vi "Parse Constructor String.vi"(11 "Input":string) -> (0 "error out":errorcluster, 3 "Result":T1)   [LabVIEW 2020, in "Stream.lvlib" / "URLPattern.lvclass"]
uses:
  URLPattern.lvclass
  URL Pattern Init.ctl
  Tokenize Policy.ctl
  Token Type.ctl
  Parser State.ctl
  Is Non-Special Pattern Char.vi
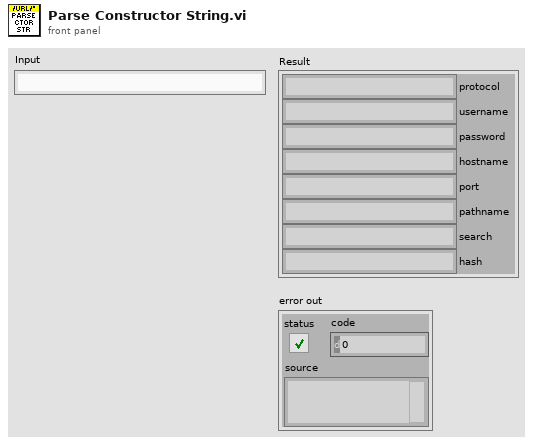
[diagram p1: front panel]
types:
  T1 = typedef "Stream.lvlib/URLPattern.lvclass/URL Pattern Init.ctl" = cluster{"protocol":string, "username":string, "password":string, "hostname":string, "port":string, "pathname":string, "search":string, "hash":string}
  T2 = typedef "Stream.lvlib/URLPattern.lvclass/Tokenize Policy.ctl" = enum16{"strict", "lenient"}
  T3 = typedef "Stream.lvlib/URLPattern.lvclass/Token.ctl" = cluster{"Type":T4, "Index":i32, "Value":string}
  T4 = typedef "Stream.lvlib/URLPattern.lvclass/Token Type.ctl" = enum16{"invalid-char", "open", "close", "regexp", "name", "char", "escaped-char", "other-modifier", "asterisk", "end"}
  T5 = typedef "Stream.lvlib/URLPattern.lvclass/Constructor String Parser.ctl" = cluster{"Input":string, "Token List":T3[], "Result":T1, "Component Start":i32, "Token Index":i32, "Token Increment":i32, "Group Depth":i32, "Hostname IPv6 Bracket Depth":i32, "Protocol Matches Special Scheme":bool, "State":T6, "List Length":i32}
  T6 = typedef "Stream.lvlib/URLPattern.lvclass/Parser State.ctl" = enum16{"init", "protocol", "authority", "username", "password", "hostname", "port", "pathname", "search", "hash", "done"}
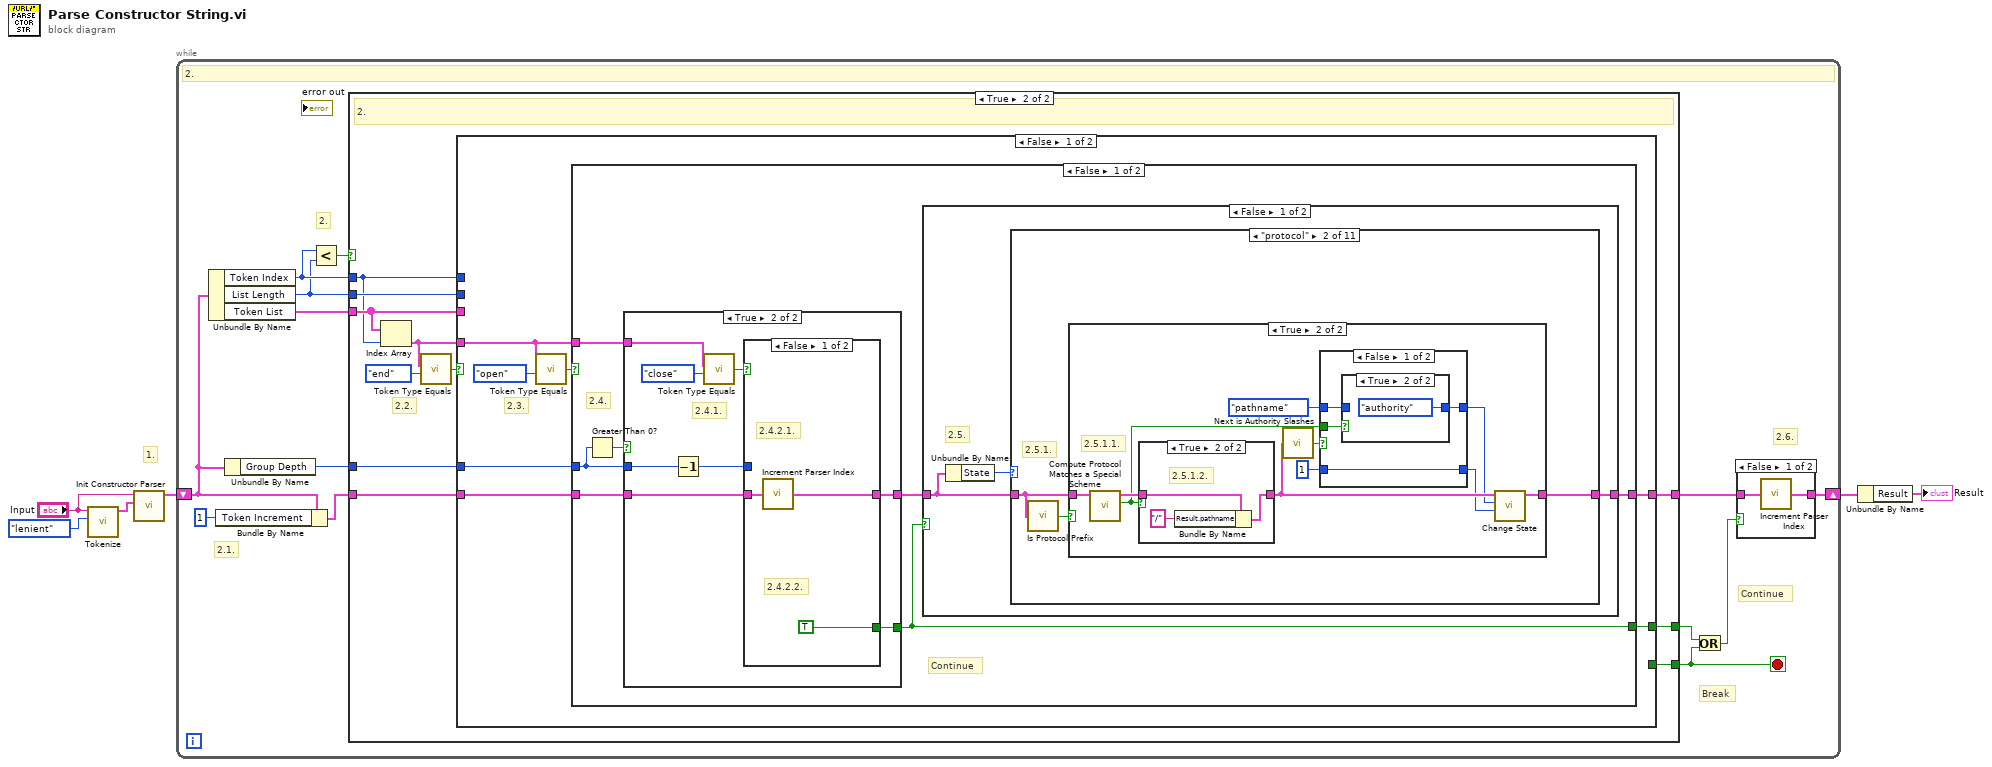
[diagram p0: block diagram]
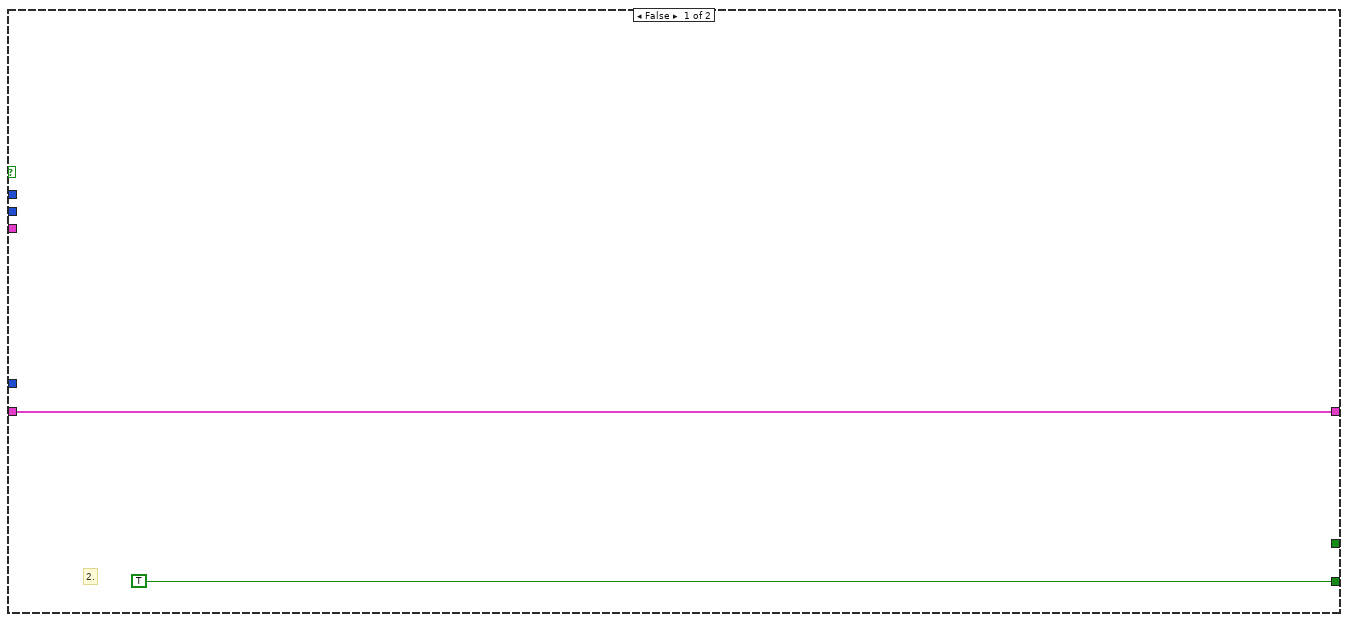
[diagram p2: hidden frame]
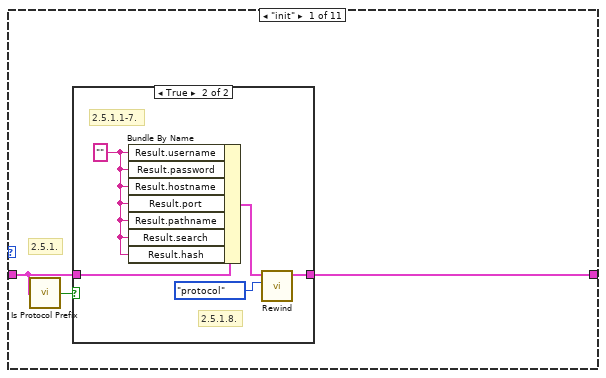
[diagram p3: hidden frame]
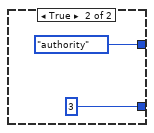
[diagram p7: hidden frame]
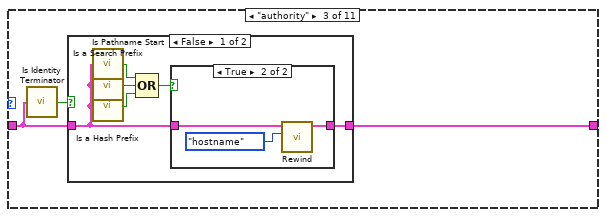
[diagram p9: hidden frame]
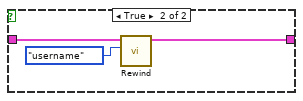
[diagram p11: hidden frame]
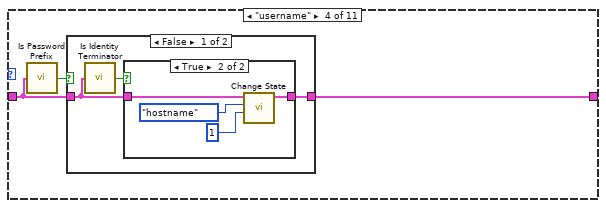
[diagram p12: hidden frame]
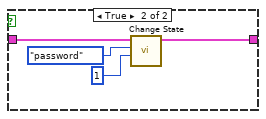
[diagram p14: hidden frame]
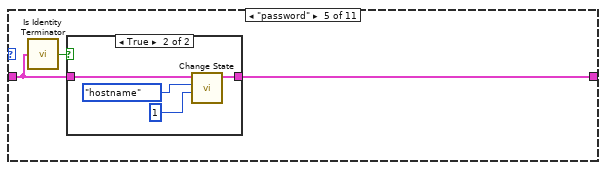
[diagram p15: hidden frame]
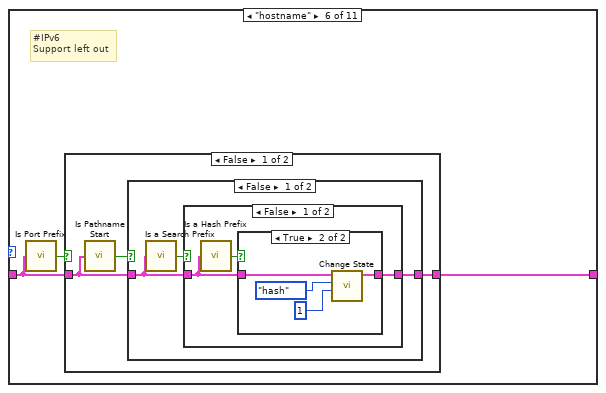
[diagram p17: hidden frame]
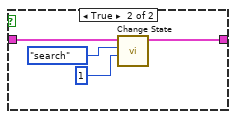
[diagram p19: hidden frame]
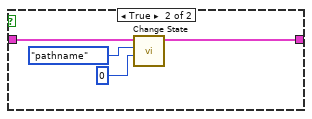
[diagram p20: hidden frame]
diagram:
  # "1."
  n1 = call "Tokenize.vi"("Policy"=Tokenize_Policy."lenient", "Input"="Input") -> ("Token List"=w4:T3[])  [unwired: 8 in, 1 out]
  n2 = call "Init Constructor Parser.vi"("Token List"=w4, "Input"="Input") -> ("Constructor String Parser"=w3:T5)  [unwired: 9 in]
  n3 = while {
    shift-right: [w11] -> w2
    shift-left: w3 -> [w8]
    stop <- w9 stop-if-true
    # "2.6."
    # "Break"
    # "Continue"
    # "2.1."
    # "2."
    # "2."
    n4 = Unbundle By Name(w8) -> ("Token Index"=w15:i32, "List Length"=w14:i32, "Token List"=w16:T3[])
    n5 = Bundle By Name(cluster=w8, "Token Increment"=1) -> (w17:T5)
    n6 = Unbundle By Name(w8) -> ("Group Depth"=w7:i32)
    n7 = Less?(x=w15, y=w14) -> (x < y?=w19:bool)
    n8 = case shown="True" w19 {
      tunnel: [TRUE w24] -> w9
      tunnel: w17 -> [w20 w30]
      tunnel: w16 -> [_ w28]
      tunnel: w15 -> [_ w26]
      tunnel: w14 -> [_ w27]
      tunnel: [w20 w25] -> w12
      tunnel: [_ w23] -> w13
      tunnel: w7 -> [_ w22]
      frame False {
        # "2."
      }
      frame True {
        # "2.2."
        # "2."
        n9 = Index Array(array=w28, index=w26) -> (element=w29:T3)
        n10 = call "Token Type Equals.vi"("Type"=Token_Type."end", "Token"=w29) -> ("Type Equals?"=w31:bool)  [unwired: 2 in]
        n11 = case shown="False" w31 {
          tunnel: w30 -> [w36 w232]
          tunnel: w29 -> [w38 _]
          tunnel: w28 -> [_ _]
          tunnel: w27 -> [_ _]
          tunnel: w26 -> [_ _]
          tunnel: [w35 w229] -> w25
          tunnel: [_ w228] -> w24
          tunnel: [w34 w227] -> w23
          tunnel: w22 -> [w33 _]
          frame False {
            # "2.3."
            n12 = call "Token Type Equals.vi"("Type"=Token_Type."open", "Token"=w38) -> ("Type Equals?"=w37:bool)  [unwired: 2 in]
            n13 = case shown="False" w37 {
              tunnel: w38 -> [w46 _]
              tunnel: w36 -> [w43 w221]
              tunnel: [w40 w219] -> w35
              tunnel: [w42 TRUE] -> w34
              tunnel: w33 -> [w44 _]
              frame False {
                # "Continue"
                # "2.4."
                n14 = Greater Than 0?(x=w44) -> (x > 0?=w45:bool)
                n15 = case shown="True" w45 {
                  tunnel: w46 -> [_ w210]
                  tunnel: w44 -> [_ w205]
                  tunnel: w43 -> [w203 w208]
                  tunnel: [w203 w207] -> w41
                  tunnel: [_ w206] -> w42
                  frame False {
                  }
                  frame True {
                    # "2.4.1."
                    n16 = Decrement(x=w205) -> (x-1=w204:i32)
                    n17 = call "Token Type Equals.vi"("Type"=Token_Type."close", "Token"=w210) -> ("Type Equals?"=w209:bool)  [unwired: 2 in]
                    n18 = case shown="False" w209 {
                      tunnel: w208 -> [w214 w217]
                      tunnel: [w213 w216] -> w207
                      tunnel: [TRUE _] -> w206
                      tunnel: w204 -> [_ w215]
                      frame False {
                        # "2.4.2.2."
                        # "2.4.2.1."
                        n19 = call "Increment Parser Index.vi"("Constructor String Parser In"=w214) -> ("Constructor String Parser"=w213:T5)
                      }
                      frame True {
                        # "2.4.1."
                        n20 = Bundle By Name(cluster=w217, "Group Depth"=w215) -> (w216:T5)
                      }
                    }
                  }
                }
                n21 = case shown="False" w42 {
                  tunnel: w41 -> [w48 w202]
                  tunnel: [w47 w202] -> w40
                  frame False {
                    # "2.5."
                    n22 = Unbundle By Name(w48) -> ("State"=w49:T6)
                    n23 = case shown="\"protocol\"" w49 {
                      tunnel: w48 -> [w51 w61 w87 w102 w117 w125 w154 w176 w191 w198 w201]
                      tunnel: [w52 w59 w85 w101 w116 w124 w153 w175 w190 w198 w201] -> w47
                      frame "init" {
                        # "2.5.1."
                        n24 = call "Is Protocol Prefix.vi"("Constructor String Parser"=w51) -> ("Is Protocol Prefix?"=w50:bool)
                        n25 = case shown="True" w50 {
                          tunnel: w51 -> [w53 w58]
                          tunnel: [w53 w56] -> w52
                          frame False {
                          }
                          frame True {
                            w57 = "" ("Result.username")
                            # "2.5.1.8."
                            # "2.5.1.1-7."
                            n26 = Bundle By Name(cluster=w58, "Result.username"=w57, "Result.password"=w57, "Result.hostname"=w57, "Result.port"=w57, "Result.pathname"=w57, "Result.search"=w57, "Result.hash"=w57) -> (w55:T5)
                            n27 = call "Rewind.vi"("State (No Change)"=Parser_State."protocol", "Constructor String Parser In"=w55) -> ("Constructor String Parser"=w56:T5)  [unwired: 9 in]
                          }
                        }
                      }
                      frame "protocol" {
                        # "2.5.1."
                        n28 = call "Is Protocol Prefix.vi"("Constructor String Parser"=w61) -> ("Is Protocol Prefix?"=w60:bool)
                        n29 = case shown="True" w60 {
                          tunnel: w61 -> [w62 w72]
                          tunnel: [w62 w63] -> w59
                          frame False {
                          }
                          frame True {
                            # "2.5.1.1."
                            n30 = call "Compute Protocol Matches a Special Scheme.vi"("Constructor String Parser In"=w72) -> ("Special Scheme"=w69:bool, "Constructor String Parser"=w71:T5)  [unwired: 8 in, 1 out]
                            n31 = case shown="True" w69 {
                              tunnel: w71 -> [w81 w84]
                              tunnel: [w81 w82] -> w66
                              frame False {
                              }
                              frame True {
                                # "2.5.1.2."
                                n32 = Bundle By Name(cluster=w84, "Result.pathname"="/") -> (w82:T5)
                              }
                            }
                            n33 = call "Next is Authority Slashes.vi"("Constructor String Parser"=w66) -> ("Authority Slashes"=w70:bool)
                            n34 = case shown="False" w70 {
                              tunnel: w69 -> [w76 _]
                              tunnel: 1 -> [w74 _]
                              tunnel: Parser_State."pathname" ("Parser State") -> [w75 _]
                              tunnel: [w74 3] -> w64
                              tunnel: [w73 Parser_State."authority" ("Parser State")] -> w65
                              frame False {
                                n35 = case shown="True" w76 {
                                tunnel: w75 -> [w77 _]
                                tunnel: [w77 Parser_State."authority" ("Parser State")] -> w73
                                frame False {
                                }
                                frame True {
                                }
                                }
                              }
                              frame True {
                              }
                            }
                            n36 = call "Change State.vi"("Skip"=w64, "New State"=w65, "Constructor String Parser In"=w66) -> ("Constructor String Parser"=w63:T5)  [unwired: 8 in]
                          }
                        }
                      }
                      frame "authority" {
                        n37 = call "Is Identity Terminator.vi"("Constructor String Parser"=w87) -> ("Is Identity Terminator"=w86:bool)
                        n38 = case shown="False" w86 {
                          tunnel: w87 -> [w90 w100]
                          tunnel: [w88 w98] -> w85
                          frame False {
                            n39 = call "Is Pathname Start.vi"("Constructor String Parser"=w90) -> ("Is Pathname Start"=w92:bool)
                            n40 = call "Is a Search Prefix.vi"("Constructor String Parser"=w90) -> ("Is a Search Prefix?"=w93:bool)
                            n41 = call "Is a Hash Prefix.vi"("Constructor String Parser"=w90) -> ("Is a Hash Prefix?"=w91:bool)
                            n42 = Compound Arithmetic op=OR(w92, w93, w91) -> (w89:bool)
                            n43 = case shown="True" w89 {
                              tunnel: w90 -> [w94 w97]
                              tunnel: [w94 w95] -> w88
                              frame False {
                              }
                              frame True {
                                n44 = call "Rewind.vi"("State (No Change)"=Parser_State."hostname", "Constructor String Parser In"=w97) -> ("Constructor String Parser"=w95:T5)  [unwired: 9 in]
                              }
                            }
                          }
                          frame True {
                            n45 = call "Rewind.vi"("State (No Change)"=Parser_State."username", "Constructor String Parser In"=w100) -> ("Constructor String Parser"=w98:T5)  [unwired: 9 in]
                          }
                        }
                      }
                      frame "username" {
                        n46 = call "Is Password Prefix.vi"("Constructor String Parser"=w102) -> ("Is Password Prefix?"=w103:bool)
                        n47 = case shown="False" w103 {
                          tunnel: w102 -> [w105 w115]
                          tunnel: [w104 w112] -> w101
                          frame False {
                            n48 = call "Is Identity Terminator.vi"("Constructor String Parser"=w105) -> ("Is Identity Terminator"=w106:bool)
                            n49 = case shown="True" w106 {
                              tunnel: w105 -> [w107 w111]
                              tunnel: [w107 w110] -> w104
                              frame False {
                              }
                              frame True {
                                n50 = call "Change State.vi"("Skip"=1, "New State"=Parser_State."hostname", "Constructor String Parser In"=w111) -> ("Constructor String Parser"=w110:T5)  [unwired: 8 in]
                              }
                            }
                          }
                          frame True {
                            n51 = call "Change State.vi"("Skip"=1, "New State"=Parser_State."password", "Constructor String Parser In"=w115) -> ("Constructor String Parser"=w112:T5)  [unwired: 8 in]
                          }
                        }
                      }
                      frame "password" {
                        n52 = call "Is Identity Terminator.vi"("Constructor String Parser"=w117) -> ("Is Identity Terminator"=w118:bool)
                        n53 = case shown="True" w118 {
                          tunnel: w117 -> [w119 w123]
                          tunnel: [w119 w120] -> w116
                          frame False {
                          }
                          frame True {
                            n54 = call "Change State.vi"("Skip"=1, "New State"=Parser_State."hostname", "Constructor String Parser In"=w123) -> ("Constructor String Parser"=w120:T5)  [unwired: 8 in]
                          }
                        }
                      }
                      frame "hostname" {
                        # "#IPv6\nSupport left out"
                        n55 = call "Is Port Prefix.vi"("Constructor String Parser"=w125) -> ("Is Port Prefix?"=w126:bool)
                        n56 = case shown="False" w126 {
                          tunnel: w125 -> [w128 w152]
                          tunnel: [w127 w149] -> w124
                          frame False {
                            n57 = call "Is Pathname Start.vi"("Constructor String Parser"=w128) -> ("Is Pathname Start"=w129:bool)
                            n58 = case shown="False" w129 {
                              tunnel: w128 -> [w131 w148]
                              tunnel: [w130 w145] -> w127
                              frame False {
                                n59 = call "Is a Search Prefix.vi"("Constructor String Parser"=w131) -> ("Is a Search Prefix?"=w132:bool)
                                n60 = case shown="False" w132 {
                                tunnel: w131 -> [w134 w144]
                                tunnel: [w133 w141] -> w130
                                frame False {
                                n61 = call "Is a Hash Prefix.vi"("Constructor String Parser"=w134) -> ("Is a Hash Prefix?"=w135:bool)
                                n62 = case shown="True" w135 {
                                tunnel: w134 -> [w136 w140]
                                tunnel: [w136 w139] -> w133
                                frame False {
                                }
                                frame True {
                                n63 = call "Change State.vi"("Skip"=1, "New State"=Parser_State."hash", "Constructor String Parser In"=w140) -> ("Constructor String Parser"=w139:T5)  [unwired: 8 in]
                                }
                                }
                                }
                                frame True {
                                n64 = call "Change State.vi"("Skip"=1, "New State"=Parser_State."search", "Constructor String Parser In"=w144) -> ("Constructor String Parser"=w141:T5)  [unwired: 8 in]
                                }
                                }
                              }
                              frame True {
                                n65 = call "Change State.vi"("Skip"=0, "New State"=Parser_State."pathname", "Constructor String Parser In"=w148) -> ("Constructor String Parser"=w145:T5)  [unwired: 8 in]
                              }
                            }
                          }
                          frame True {
                            n66 = call "Change State.vi"("Skip"=1, "New State"=Parser_State."port", "Constructor String Parser In"=w152) -> ("Constructor String Parser"=w149:T5)  [unwired: 8 in]
                          }
                        }
                      }
                      frame "port" {
                        n67 = call "Is Pathname Start.vi"("Constructor String Parser"=w154) -> ("Is Pathname Start"=w155:bool)
                        n68 = case shown="False" w155 {
                          tunnel: w154 -> [w157 w174]
                          tunnel: [w156 w171] -> w153
                          frame False {
                            n69 = call "Is a Search Prefix.vi"("Constructor String Parser"=w157) -> ("Is a Search Prefix?"=w158:bool)
                            n70 = case shown="False" w158 {
                              tunnel: w157 -> [w160 w170]
                              tunnel: [w159 w167] -> w156
                              frame False {
                                n71 = call "Is a Hash Prefix.vi"("Constructor String Parser"=w160) -> ("Is a Hash Prefix?"=w161:bool)
                                n72 = case shown="True" w161 {
                                tunnel: w160 -> [w162 w166]
                                tunnel: [w162 w165] -> w159
                                frame False {
                                }
                                frame True {
                                n73 = call "Change State.vi"("Skip"=1, "New State"=Parser_State."hash", "Constructor String Parser In"=w166) -> ("Constructor String Parser"=w165:T5)  [unwired: 8 in]
                                }
                                }
                              }
                              frame True {
                                n74 = call "Change State.vi"("Skip"=1, "New State"=Parser_State."search", "Constructor String Parser In"=w170) -> ("Constructor String Parser"=w167:T5)  [unwired: 8 in]
                              }
                            }
                          }
                          frame True {
                            n75 = call "Change State.vi"("Skip"=0, "New State"=Parser_State."pathname", "Constructor String Parser In"=w174) -> ("Constructor String Parser"=w171:T5)  [unwired: 8 in]
                          }
                        }
                      }
                      frame "pathname" {
                        n76 = call "Is a Search Prefix.vi"("Constructor String Parser"=w176) -> ("Is a Search Prefix?"=w177:bool)
                        n77 = case shown="False" w177 {
                          tunnel: w176 -> [w179 w189]
                          tunnel: [w178 w186] -> w175
                          frame False {
                            n78 = call "Is a Hash Prefix.vi"("Constructor String Parser"=w179) -> ("Is a Hash Prefix?"=w180:bool)
                            n79 = case shown="True" w180 {
                              tunnel: w179 -> [w181 w185]
                              tunnel: [w181 w184] -> w178
                              frame False {
                              }
                              frame True {
                                n80 = call "Change State.vi"("Skip"=1, "New State"=Parser_State."hash", "Constructor String Parser In"=w185) -> ("Constructor String Parser"=w184:T5)  [unwired: 8 in]
                              }
                            }
                          }
                          frame True {
                            n81 = call "Change State.vi"("Skip"=1, "New State"=Parser_State."search", "Constructor String Parser In"=w189) -> ("Constructor String Parser"=w186:T5)  [unwired: 8 in]
                          }
                        }
                      }
                      frame "search" {
                        n82 = call "Is a Hash Prefix.vi"("Constructor String Parser"=w191) -> ("Is a Hash Prefix?"=w192:bool)
                        n83 = case shown="True" w192 {
                          tunnel: w191 -> [w193 w197]
                          tunnel: [w193 w194] -> w190
                          frame False {
                          }
                          frame True {
                            n84 = call "Change State.vi"("Skip"=1, "New State"=Parser_State."hash", "Constructor String Parser In"=w197) -> ("Constructor String Parser"=w194:T5)  [unwired: 8 in]
                          }
                        }
                      }
                      frame "hash" {
                      }
                      frame "done" {
                        # "#ASSERT\nShould never get here."
                        n85 = call <vilib>:"Simple Error Handler.vi"("error code (no error:0)"=-2132869109, "error source (\" \")"="Failed Assert, should never reach done state." ("error source (\" \")")) -> ()  [unwired: 3 in, 5 out]
                      }
                    }
                  }
                  frame True {
                  }
                }
              }
              frame True {
                # "2.3.3."
                # "2.3.2."
                # "2.3.1."
                n86 = Unbundle By Name(w221) -> ("Token Increment"=w220:i32)
                n87 = in-place {
                  in-place-border: w220 -> [w222]
                  n88 = in-place-cluster #1(w221) -> ("Group Depth"=w226:i32, "Token Index"=w224:i32)
                  n89 = Increment(x=w226) -> (x+1=w225:i32)
                  n90 = Add(x=w224, y=w222) -> (x+y=w223:i32)
                  n91 = in-place-cluster #1("Group Depth"=w225, "Token Index"=w223) -> (w219:T5)
                }
              }
            }
          }
          frame True {
            # "Continue?"
            # "2.2.1."
            n92 = call "Parser State Equals.vi"("State"=Parser_State."init", "Constructor String Parser"=w232) -> ("State Equals?"=w233:bool)  [unwired: 2 in]
            n93 = case shown="False" w233 {
              tunnel: w232 -> [w244 w258]
              tunnel: [w243 w254] -> w231
              tunnel: [w242 TRUE] -> w230
              frame False {
                # "2.2.2."
                # "2.2.2."
                n94 = call "Parser State Equals.vi"("State"=Parser_State."authority", "Constructor String Parser"=w244) -> ("State Equals?"=w245:bool)  [unwired: 2 in]
                n95 = case shown="True" w245 {
                  tunnel: w244 -> [w247 w252]
                  tunnel: [w247 w249] -> w243
                  tunnel: [_ TRUE] -> w242
                  frame False {
                  }
                  frame True {
                    # "2.2.2.3."
                    # "2.2.2.2."
                    # "2.2.2.1."
                    n96 = call "Rewind.vi"("State (No Change)"=Parser_State."hostname", "Constructor String Parser In"=w252) -> ("Constructor String Parser"=w250:T5)  [unwired: 9 in]
                    n97 = call "Increment Parser Index.vi"("Constructor String Parser In"=w250) -> ("Constructor String Parser"=w249:T5)
                  }
                }
              }
              frame True {
                # "2.2.1.6."
                # "2.2.1.5."
                # "2.2.1.2."
                # "2.2.1.1."
                # "2.2.1.1."
                n98 = call "Rewind.vi"("Constructor String Parser In"=w258) -> ("Constructor String Parser"=w256:T5)  [unwired: 10 in]
                n99 = call "Is a Hash Prefix.vi"("Constructor String Parser"=w256) -> ("Is a Hash Prefix?"=w257:bool)
                n100 = case shown="False" w257 {
                  tunnel: w256 -> [w260 w281]
                  tunnel: [w259 w278] -> w255
                  frame False {
                    # "2.2.1.3."
                    # "2.2.1.3."
                    n101 = call "Is a Search Prefix.vi"("Constructor String Parser"=w260) -> ("Is a Search Prefix?"=w261:bool)
                    n102 = case shown="False" w261 {
                      tunnel: w260 -> [w270 w277]
                      tunnel: [w262 w271] -> w259
                      frame False {
                        w263 = "" ("Result")
                        # "2.2.1.4.3."
                        # "2.2.1.4.2."
                        # "2.2.1.4.1."
                        # "2.2.1.4."
                        n103 = call "Change State.vi"("Skip"=0, "New State"=Parser_State."pathname", "Constructor String Parser In"=w270) -> ("Constructor String Parser"=w267:T5)  [unwired: 8 in]
                        n104 = call "Set Parser Result.vi"("Result"=w263, "State"=Parser_State."search", "Constructor String Parser In"=w267) -> ("Constructor String Parser"=w265:T5)  [unwired: 8 in]
                        n105 = call "Set Parser Result.vi"("Result"=w263, "State"=Parser_State."hash", "Constructor String Parser In"=w265) -> ("Constructor String Parser"=w262:T5)  [unwired: 8 in]
                      }
                      frame True {
                        # "2.2.1.3.2."
                        # "2.2.1.3.1."
                        # "2.2.1.3."
                        n106 = call "Change State.vi"("Skip"=1, "New State"=Parser_State."search", "Constructor String Parser In"=w277) -> ("Constructor String Parser"=w274:T5)  [unwired: 8 in]
                        n107 = call "Set Parser Result.vi"("Result"="", "State"=Parser_State."hash", "Constructor String Parser In"=w274) -> ("Constructor String Parser"=w271:T5)  [unwired: 8 in]
                      }
                    }
                  }
                  frame True {
                    # "2.2.1.2."
                    n108 = call "Change State.vi"("Skip"=1, "New State"=Parser_State."hash", "Constructor String Parser In"=w281) -> ("Constructor String Parser"=w278:T5)  [unwired: 8 in]
                  }
                }
                n109 = call "Increment Parser Index.vi"("Constructor String Parser In"=w255) -> ("Constructor String Parser"=w254:T5)
              }
            }
            n110 = case shown="False" w230 {
              selector: w230 -> [_ w240]
              tunnel: w231 -> [w239 w241]
              tunnel: [w237 w241] -> w229
              tunnel: [TRUE _] -> w228
              tunnel: [_ w240] -> w227
              frame False {
                # "2.2.4."
                n111 = call "Change State.vi"("Skip"=0, "New State"=Parser_State."done", "Constructor String Parser In"=w239) -> ("Constructor String Parser"=w237:T5)  [unwired: 8 in]
              }
              frame True {
              }
            }
          }
        }
      }
    }
    n112 = Or(x=w13, y=w9) -> (x .or. y?=w10:bool)
    n113 = case shown="False" w10 {
      tunnel: w12 -> [w283 w284]
      tunnel: [w282 w284] -> w11
      frame False {
        n114 = call "Increment Parser Index.vi"("Constructor String Parser In"=w283) -> ("Constructor String Parser"=w282:T5)
      }
      frame True {
      }
    }
  }
  n115 = Unbundle By Name(w2) -> ("Result"=→"Result":T1)
